vi "Get Matrix String.vi"(10 "matrix key":string, 11 "info data":string) -> (1 "exist":bool, 3 "matrix part":string)   [LabVIEW 2013, in "infolib.lvlib"]
doc: "Finds section structure and return its content. If not found, exist is false. If no section structure set, returns whole info data and exist is true."
uses:
  infolib.lvlib
  <vilib>/regexp/Match Regular Expression.xnode
panel:
  out "regexp":string
  # "testing string: (put \"1\" and \"2\" into section names)"
  # "blfdablad\n#startmatrix:: a\n1; 2; 3;\n#endmatrix:: a\n#startsection:: 1\n   #startmatrix:: b\n   1; 2; 3;\n  4;   5 ; 6   ;\n   #endmatrix:: b\n#endsection:: 1\njfdklajfkdl"
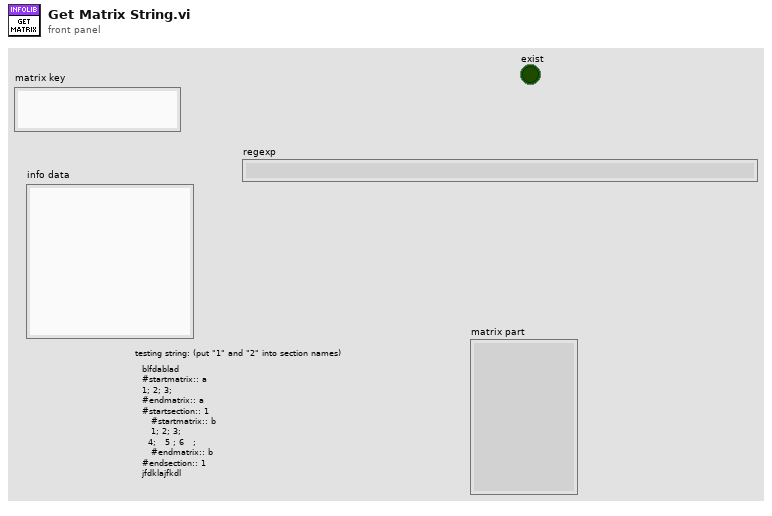
[diagram p1: front panel]
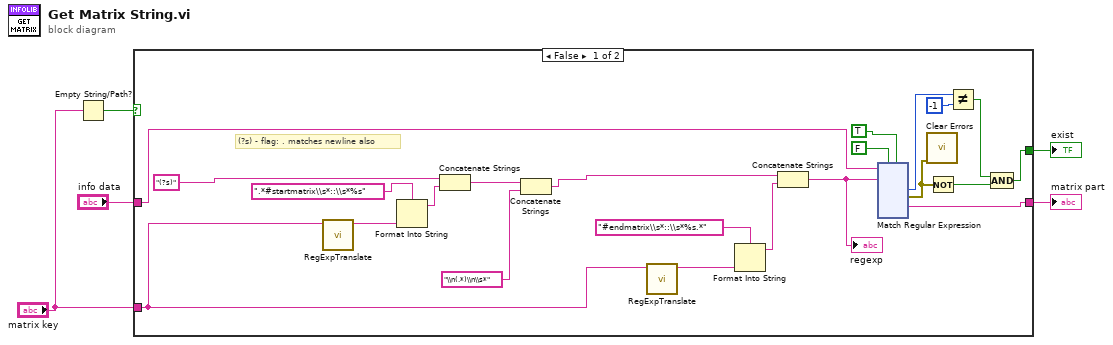
[diagram p0: block diagram]
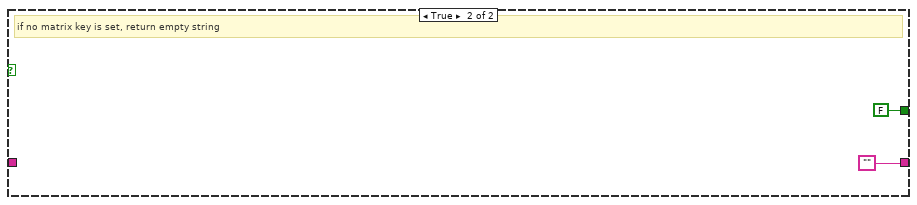
[diagram p2: hidden frame]
diagram:
  n1 = Empty String/Path?(string/path="matrix key") -> (empty?=w3:bool)
  n2 = case shown="False" w3 {
    tunnel: [w19 FALSE] -> w5
    tunnel: [w14 ""] -> w4
    tunnel: "info data" -> [w13 _]
    tunnel: "matrix key" -> [w12 _]
    frame False {
      # "(?s) - flag: . matches newline also"
      n3 = call "RegExpTranslate.vi"("string"=w12) -> ("regexp safe string"=w9:string)  [unwired: 10 in]
      n4 = Format Into String(format string=".*#startmatrix\\s*::\\s*%s", w9) -> (resulting string=w10:string)  [unwired: 2 in, 1 out]
      n5 = Concatenate Strings("(?s)" ("section name"), w10) -> (w22:string)
      n6 = Concatenate Strings(w22, "\\n(.*)\\n\\s*" ("string")) -> (w20:string)
      n7 = call "RegExpTranslate.vi"("string"=w12) -> ("regexp safe string"=w6:string)  [unwired: 10 in]
      n8 = Format Into String(format string="#endmatrix\\s*::\\s*%s.*", w6) -> (resulting string=w7:string)  [unwired: 2 in, 1 out]
      n9 = Concatenate Strings(w20, w7) -> (w15:string)
      "regexp" <- w15
      n10 = xnode "Match Regular Expression"("input string"=w13, "regular expression"=w15, "ignore case? (F)"=FALSE, "multiline? (F)"=TRUE) -> ("offset past match"=w24:i32, "error out"=w16:errorcluster, "submatch 1"=w14:string)  [unwired: 2 in, 4 out]
      n11 = call <vilib>:"Clear Errors.vi"("error in (no error)"=w16) -> ()  [unwired: 6 in, 1 out]
      n12 = Not(x=w16) -> (.not. x?=w17:bool)
      n13 = Not Equal?(x=w24, y=-1 ("x")) -> (x != y?=w18:bool)
      n14 = Compound Arithmetic op=AND(w18, w17) -> (w19:bool)
    }
    frame True {
      # "if no matrix key is set, return empty string"
    }
  }
  "exist" <- w5
  "matrix part" <- w4
